vi "Write CurrentProgramNumber.vi"(8 "error in (no error)":errorcluster, 10 "CurrentProgramNumber":u32, 11 "RampProgramModel in":refnum<class "RampProgramModel.lvclass">) -> (0 "error out":errorcluster, 3 "RampProgramModel out":refnum<class "RampProgramModel.lvclass">)   [LabVIEW 2013, in "RampProgramModel.lvclass"]
uses:
  RampProgramModel.lvclass
  RampProgramModel.lvclass/RampProgramModel.ctl
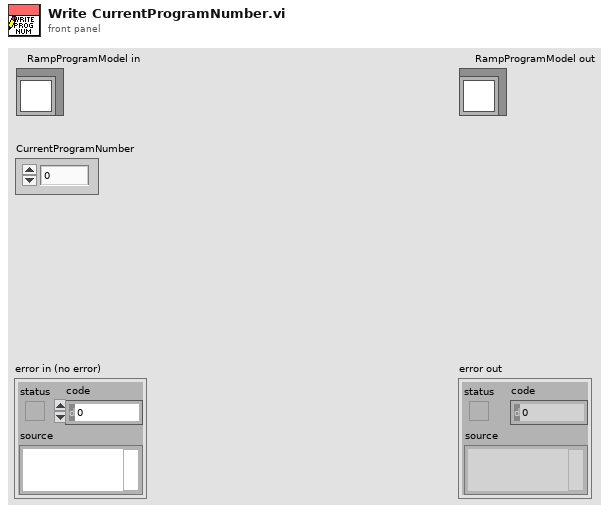
[diagram p1: front panel]
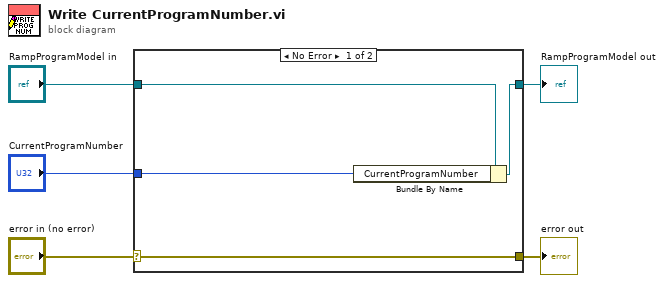
[diagram p0: block diagram]
diagram:
  n1 = case shown="No Error" "error in (no error)" {
    selector: "error in (no error)" -> [w9 w10]
    tunnel: [w9 w10] -> w4
    tunnel: [w7 w11] -> w2
    tunnel: "RampProgramModel in" -> [w8 w11]
    tunnel: "CurrentProgramNumber" -> [w6 _]
    frame No Error {
      n2 = Bundle By Name(cluster=w8, "CurrentProgramNumber"=w6) -> (w7:refnum<class "RampProgramModel.lvclass">)
    }
    frame Error {
    }
  }
  "error out" <- w4
  "RampProgramModel out" <- w2
